vi "Updatable array.vi"() -> ()   [LabVIEW 2015]
uses:
  <vilib>/Utility/miscctls.llb/LVRowAndColumnTypeDef.ctl
panel:
  out "Column 2":i32
  out "Column":i32
  out "Array":dbl[][](array[numeric])
  in  "Temp":dbl
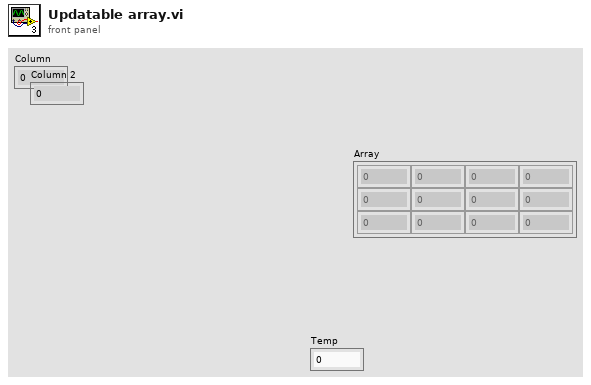
[diagram p1: front panel]
types:
  T1 = typedef "LVRowAndColumnTypeDef.ctl" = cluster{"Row":i32, "Column":i32}
  T2 = typedef "LVPoint32TypeDef.ctl" = cluster{"Horizontal":i32, "Vertical":i32}
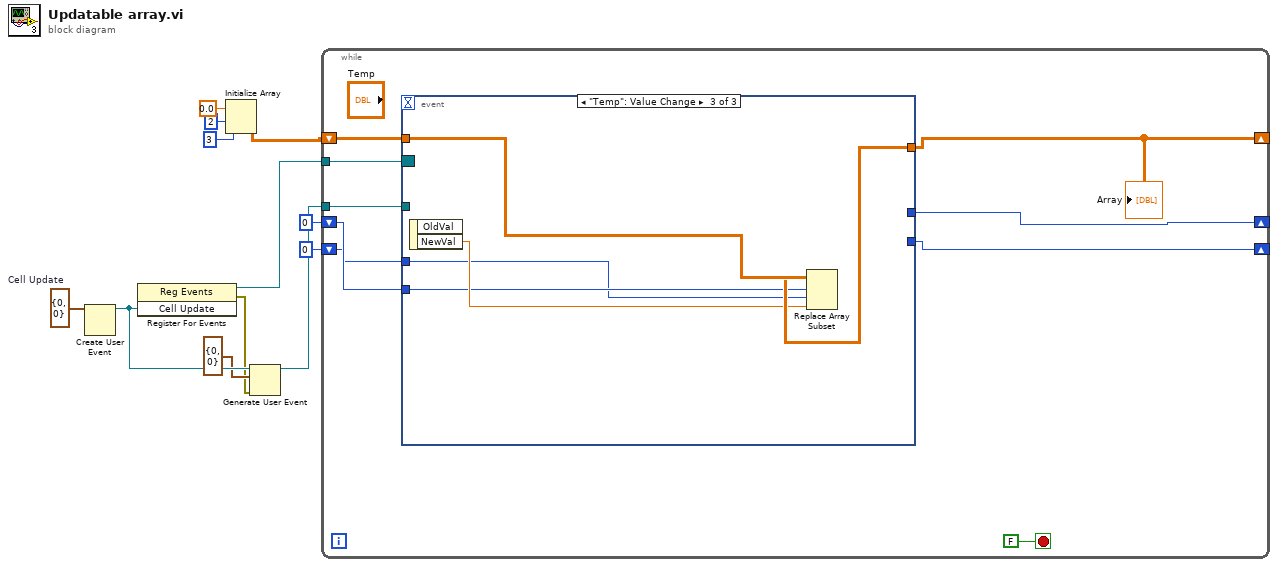
[diagram p0: block diagram]
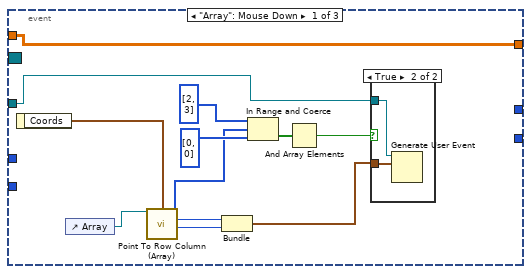
[diagram p2: hidden frame]
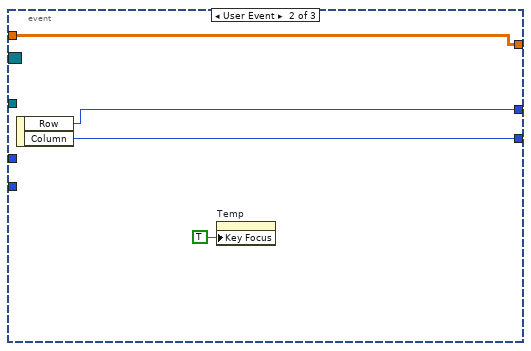
[diagram p4: hidden frame]
diagram:
  w9 = T1 {"Row"=0, "Column"=0}  # Cell Update
  n1 = Create User Event(user event datatype=w9) -> (user event=w8:refnum<user-event>)  [unwired: 1 in, 1 out]
  n2 = register-events(w8) -> (reference out=w3:refnum<event-registration>, error out=w6:errorcluster)  [unwired: 2 in]
  n3 = Initialize Array(0.0 ("element"), 2 ("dimension size"), 3 ("dimension size")) -> (w4:dbl[][])
  n4 = Generate User Event(user event=w8, event data cluster=T1 {"Row"=0, "Column"=0} ("event data"), error in=w6) -> (user event out=w5:refnum<user-event>)  [unwired: 1 in, 1 out]
  n5 = while {
    tunnel: w5 -> [w21]
    shift-right: [w19] -> _
    shift-left: w4 -> [w20]
    tunnel: w3 -> [w17]
    shift-right: [w16] -> _
    shift-left: 0 ("Row") -> [w14]
    shift-right: [w15] -> _
    shift-left: 0 ("Column") -> [w13]
    stop <- FALSE stop-if-true
    n6 = event shown="[2] \"Temp\": Value Change" {
      selector: w17 -> [_ _ _]
      dyn-events: _ -> [_ _ _]
      timeout: _ -> [_ _ _]
      tunnel: [w32 w38 w43] -> w19
      tunnel: w21 -> [w33 _ _]
      tunnel: w20 -> [w32 w38 w44]
      tunnel: [_ w37 _] -> w16
      tunnel: [_ w36 _] -> w15
      tunnel: w14 -> [_ _ w41]
      tunnel: w13 -> [_ _ w40]
      event "Array": Mouse Down {
        n7 = event-data() -> ("Coords"=w31:T2)  [unwired: 1 in]
        n8 = control-ref of="Array"() -> (w22:refnum<vi>)
        n9 = call "Point To Row Column (Array).vi"("reference"=w22, "Coords of Click"=w31) -> ("Clicked Index"=w26:i32[], "Clicked Row"=w25:i32, "Clicked Col"=w24:i32)  [unwired: 8 in, 3 out]
        n10 = Bundle("Clicked Row"=w25, "Clicked Col"=w24) -> (w23:cluster{"Clicked Row":i32, "Clicked Col":i32})  [unwired: 1 in]
        n11 = In Range and Coerce(upper limit=i32[] [2, 3], x=w26, lower limit=i32[] [0, 0]) -> (In Range?=w28:bool[])  [unwired: 1 out]
        n12 = And Array Elements(Boolean array=w28) -> (logical AND=w27:bool)
        n13 = case shown="True" w27 {
          tunnel: w33 -> [_ w35]
          tunnel: w23 -> [_ w34]
          frame False {
          }
          frame True {
            n14 = Generate User Event(user event=w35, event data cluster=w34) -> ()  [unwired: 2 in, 2 out]
          }
        }
      }
      event User Event {
        n15 = event-data() -> ("Row"=w37:i32, "Column"=w36:i32)  [unwired: 1 in]
        n16 = property on="Temp" class="DigNum (strict)"("Key Focus"=TRUE) -> ()  [unwired: 2 in, 2 out]
      }
      event "Temp": Value Change {
        n17 = event-data() -> ("NewVal"=w42:dbl)  [unwired: 1 in, 1 out]
        n18 = Replace Array Subset(array=w44, new element=w42, index (row)=w41, index (col)=w40) -> (w43:dbl[][])
      }
    }
    "Array" <- w19
  }
